vi "OTP - Create Message.vi"(7 "Keys File Path":path, 10 "Start Key":i32, 11 "message (Plain Text)":string="\"Neque porro quisquam est qui dolorem ipsum quia dolor sit amet, consectetur, adipisci velit...\"\n\"There is no one who loves pain itself, who seeks after it and wants to have it, simply because it is pain...\"") -> (3 "message (Ciphered)":string, 5 "enoughKeys?":bool)   [LabVIEW 2013]
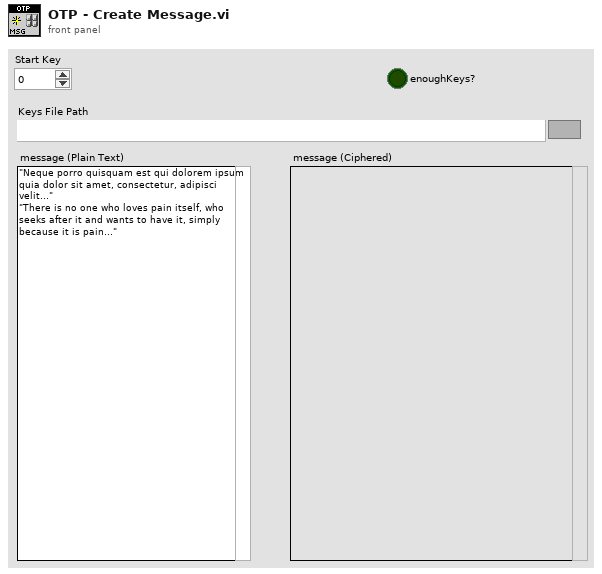
[diagram p1: front panel]
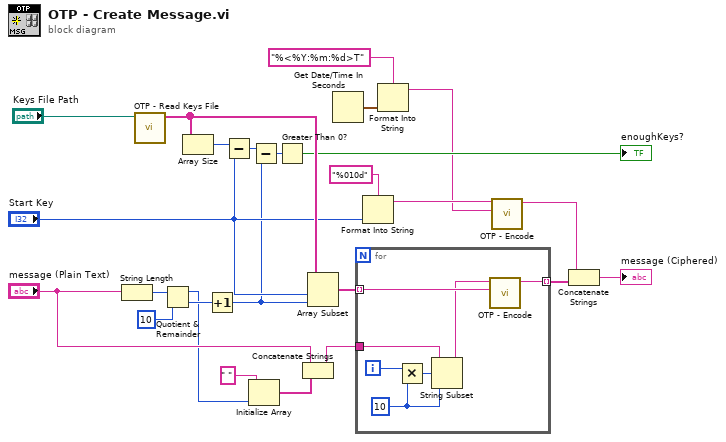
[diagram p0: block diagram]
diagram:
  n1 = String Length(string="message (Plain Text)") -> (length=w24:i32)
  n2 = call "OTP - Read Keys File.vi"("File Path"="Keys File Path") -> ("keys"=w21:string[])  [unwired: 10 in]
  n3 = Quotient & Remainder(x=w24, y=10) -> (x-y*floor(x/y)=w13:i32, floor(x/y)=w22:i32)
  n4 = Array Size(array=w21) -> (size(s)=w20:i32)
  n5 = Increment(x=w22) -> (x+1=w5:i32)
  n6 = Subtract(x=w20, y="Start Key") -> (x-y=w19:i32)
  n7 = Initialize Array(" ", w13) -> (w11:string[])
  n8 = Subtract(x=w19, y=w5) -> (x-y=w18:i32)
  n9 = Greater Than 0?(x=w18) -> (x > 0?=→"enoughKeys?":bool)
  n10 = Concatenate Strings("message (Plain Text)", w11) -> (w14:string)
  n11 = Array Subset(array=w21, index="Start Key", length=w5) -> (w16:string[])
  n12 = Get Date/Time In Seconds() -> (seconds since 1Jan1904=w3:timestamp)
  n13 = for {
    tunnel: w16 -> [w32] mode=indexing
    tunnel: w14 -> [w30]
    tunnel: [w27] -> w10 mode=indexing
    i -> [w29]
    w28 = 10 ("length (rest)")
    n14 = Multiply(x=w29, y=w28) -> (x*y=w31:i32)
    n15 = String Subset(string=w30, offset (0)=w31, length (rest)=w28) -> (substring=w26:string)
    n16 = call "OTP - Encode.vi"("Key (Private)"=w32, "message (Private)"=w26) -> ("ciphertext (Public)"=w27:string)  [unwired: 9 in]
  }
  n17 = Format Into String(format string="%010d", "Start Key") -> (resulting string=w6:string)  [unwired: 2 in, 1 out]
  n18 = Format Into String(format string="%<%Y:%m:%d>T", w3) -> (resulting string=w1:string)  [unwired: 2 in, 1 out]
  n19 = call "OTP - Encode.vi"("Key (Private)"=w1, "message (Private)"=w6) -> ("ciphertext (Public)"=w9:string)  [unwired: 9 in]
  n20 = Concatenate Strings(w9, w10) -> (→"message (Ciphered)":string)
